vi "Query Library.vi"(7 "Selection Info":T1, 8 "error in":errorcluster, 11 "Library":refnum<vi>) -> (0 "error out":errorcluster, 3 "Library Info":T1, 4 "Library Locked?":bool)   [LabVIEW 2020, in "ConstantErrorsMaker.lvlib"]
uses:
  ConstantErrorsMaker.lvlib
  Selection Info--cluster.ctl
  Selection Type--enum.ctl
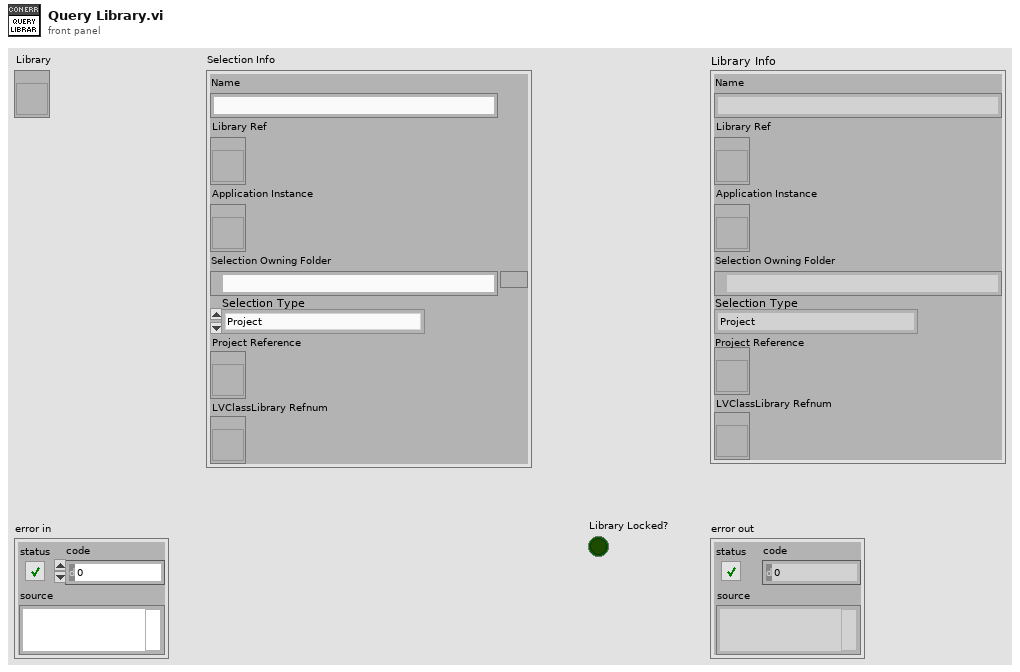
[diagram p1: front panel]
types:
  T1 = typedef "ConstantErrorsMaker.lvlib/Selection Info--cluster.ctl" = cluster{"Name":string, "Library Ref":refnum<vi>, "Application Instance":refnum<vi>, "Selection Owning Folder":path, "Selection Type":T2, "Project Reference":refnum<vi>, "LVClassLibrary Refnum":refnum<vi>}
  T2 = typedef "ConstantErrorsMaker.lvlib/Selection Type--enum.ctl" = enum16{"Project", "Library", "Class", "DQMH Singleton", "DQMH Cloneable"}
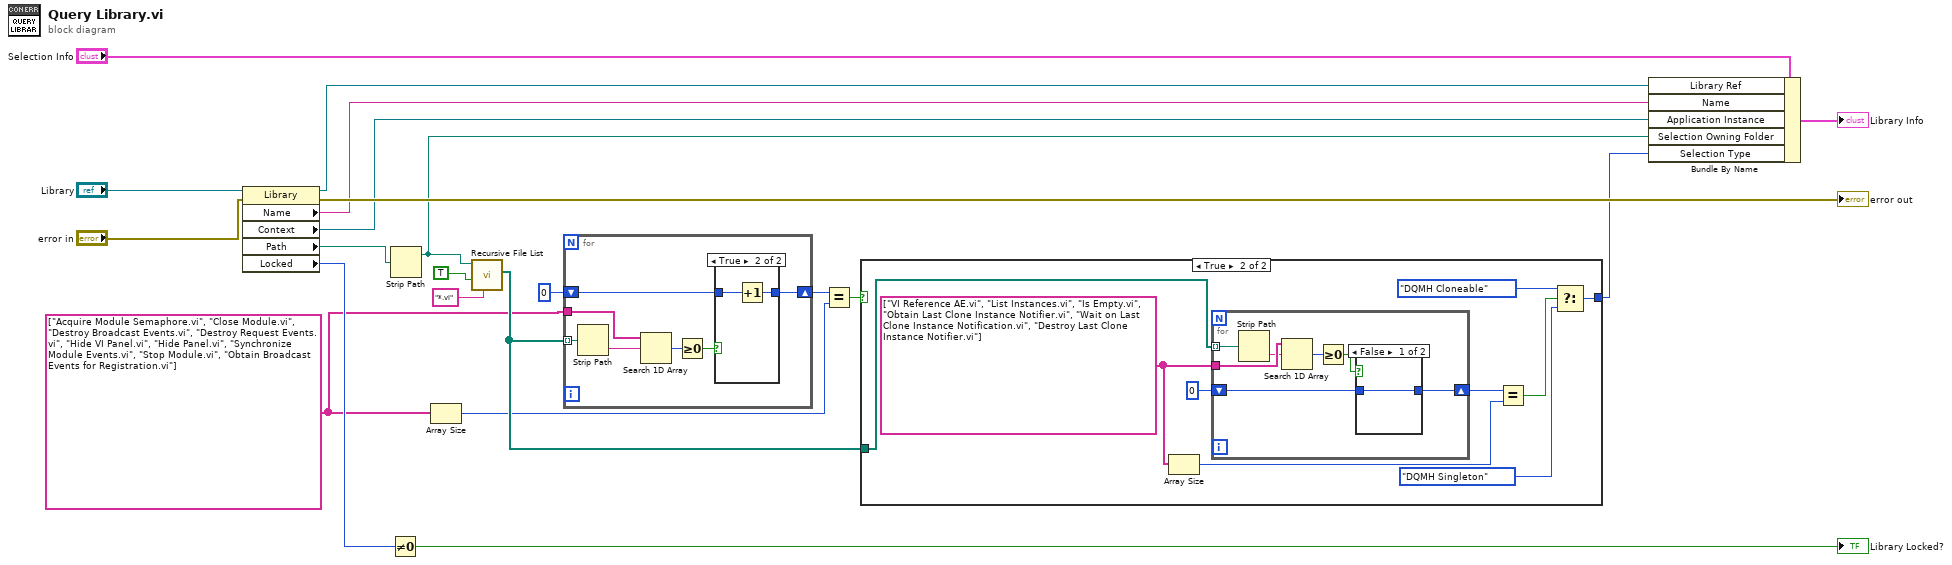
[diagram p0: block diagram]
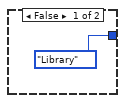
[diagram p2: hidden frame]
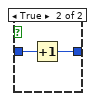
[diagram p3: hidden frame]
diagram:
  w4 = string[] ["Acquire Module Semaphore.vi", "Close Module.vi", "Destroy Broadcast Events.vi", "Destroy Request Events.vi", "Hide VI Panel.vi", "Hide Panel.vi", "Synchronize Module Events.vi", "Stop Module.vi", "Obtain Broadcast Events for Registration.vi"]
  n1 = property class="Library"(reference="Library", error in="error in") -> (reference out=w13:refnum<vi>, error out=→"error out":errorcluster, "Name"=w19:string, "Context"=w17:refnum<vi>, "Path"=w18:path, "Locked"=w16:i32)
  n2 = Not Equal To 0?(x=w16) -> (x != 0?=→"Library Locked?":bool)
  n3 = Strip Path(path=w18) -> (stripped path=w10:path)  [unwired: 1 out]
  n4 = Array Size(array=w4) -> (size(s)=w3:i32)
  n5 = call <vilib>:"Recursive File List.vi"("pattern"="*.vi", "Continue Recursing on Error? (F)"=TRUE, "Folder Path"=w10) -> ("All Files in Dir"=w7:path[])  [unwired: 4 in, 4 out]
  n6 = for {
    tunnel: w7 -> [w28] mode=indexing
    tunnel: w4 -> [w27]
    shift-right: [w22] -> w5
    shift-left: 0 -> [w23]
    n7 = Strip Path(path=w28) -> (name=w26:string)  [unwired: 1 out]
    n8 = Search 1D Array(1D array=w27, element=w26) -> (index of element=w25:i32)  [unwired: 1 in]
    n9 = Greater Or Equal To 0?(x=w25) -> (x >= 0?=w24:bool)
    n10 = case shown="True" w24 {
      tunnel: w23 -> [w29 w31]
      tunnel: [w29 w30] -> w22
      frame False {
      }
      frame True {
        n11 = Increment(x=w31) -> (x+1=w30:i32)
      }
    }
  }
  n12 = Equal?(x=w5, y=w3) -> (x = y?=w2:bool)
  n13 = case shown="True" w2 {
    tunnel: w7 -> [_ w41]
    tunnel: [Selection_Type--enum."Library" ("Selection Type") w40] -> w1
    frame False {
    }
    frame True {
      w37 = string[] ["VI Reference AE.vi", "List Instances.vi", "Is Empty.vi", "Obtain Last Clone Instance Notifier.vi", "Wait on Last Clone Instance Notification.vi", "Destroy Last Clone Instance Notifier.vi"]
      n14 = Array Size(array=w37) -> (size(s)=w36:i32)
      n15 = for {
        tunnel: w41 -> [w48] mode=indexing
        tunnel: w37 -> [w47]
        shift-right: [w42] -> w38
        shift-left: 0 -> [w43]
        n16 = Strip Path(path=w48) -> (name=w46:string)  [unwired: 1 out]
        n17 = Search 1D Array(1D array=w47, element=w46) -> (index of element=w45:i32)  [unwired: 1 in]
        n18 = Greater Or Equal To 0?(x=w45) -> (x >= 0?=w44:bool)
        n19 = case shown="False" w44 {
          tunnel: w43 -> [w49 w51]
          tunnel: [w49 w50] -> w42
          frame False {
          }
          frame True {
            n20 = Increment(x=w51) -> (x+1=w50:i32)
          }
        }
      }
      n21 = Equal?(x=w38, y=w36) -> (x = y?=w35:bool)
      n22 = Select(t=Selection_Type--enum."DQMH Cloneable" ("Selection Type"), s=w35, f=Selection_Type--enum."DQMH Singleton" ("Selection Type")) -> (s? t:f=w40:T2)
    }
  }
  n23 = Bundle By Name(cluster="Selection Info", "Library Ref"=w13, "Name"=w19, "Application Instance"=w17, "Selection Owning Folder"=w10, "Selection Type"=w1) -> (→"Library Info":T1)
